vi "Format_table.vi"(2 "Table Control":refnum<vi>) -> ()   [LabVIEW 2013]
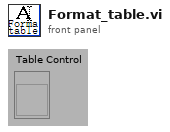
[diagram p1: front panel]
types:
  T1 = cluster{"Font Name:":string, "Size":i16, "Strikeout?":bool, "Italic?":bool, "Underline?":bool, "Outline?":bool, "Shadow?":bool, "Bold?":bool}
  T2 = enum16{"User-specified Font", "Application Font", "System Font", "Dialog Font"}
  T3 = typedef "LVFontTypeDef.ctl" = cluster{"Font Name":string, "Size":u16, "Bold":bool, "Italic":bool, "Underline":bool, "Strikeout":bool, "Color":u32}
  T4 = cluster{"left":i16, "top":i16, "right":i16, "bottom":i16}
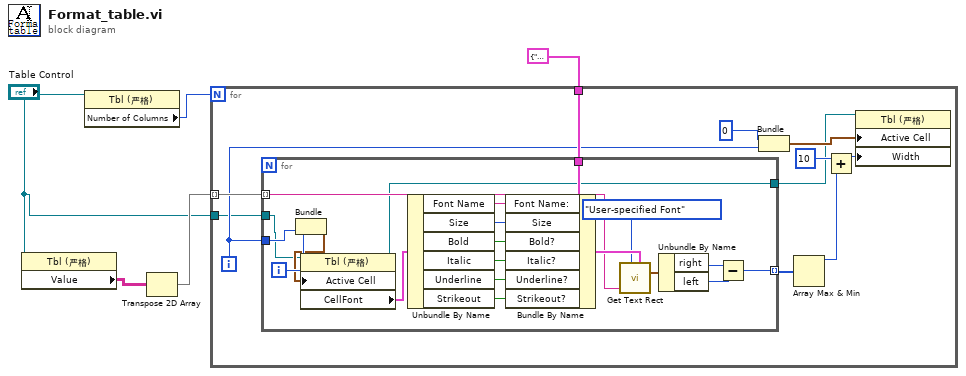
[diagram p0: block diagram]
diagram:
  n1 = property class="Tbl (严格)"(reference="Table Control") -> ("Value"=w3:string[][])  [unwired: 1 in, 2 out]
  n2 = property class="Tbl (严格)"(reference="Table Control") -> ("Number of Columns"=w2:u32)  [unwired: 1 in, 2 out]
  n3 = Transpose 2D Array(2D array=w3) -> (transposed array=w4:string[][])
  n4 = for {
    N: w2 -> [_]
    tunnel: w4 -> [w16] mode=indexing
    tunnel: T1 {"Font Name:"="", "Size"=0, "Strikeout?"=FALSE, "Italic?"=FALSE, "Underline?"=FALSE, "Outline?"=FALSE, "Shadow?"=FALSE, "Bold?"=FALSE} ("[user-specified font]") -> [w15]
    tunnel: "Table Control" -> [w7]
    i -> [w13]
    n5 = for {
      tunnel: w16 -> [w28] mode=indexing
      tunnel: w13 -> [w21]
      tunnel: w15 -> [w35]
      tunnel: [w23] -> w14 mode=indexing
      tunnel: w7 -> [w18]
      tunnel: [w17] -> w6
      i -> [w22]
      n6 = Bundle(w22, w21) -> (w20:cluster{i32, i32})  [unwired: 1 in]
      n7 = property class="Tbl (严格)"(reference=w18, "Active Cell"=w20) -> (reference out=w17:refnum<vi>, "CellFont"=w19:T3)  [unwired: 1 in, 1 out]
      n8 = Unbundle By Name(w19) -> ("Font Name"=w34:string, "Size"=w33:u16, "Bold"=w32:bool, "Italic"=w31:bool, "Underline"=w30:bool, "Strikeout"=w29:bool)
      n9 = Bundle By Name(cluster=w35, "Font Name:"=w34, "Size"=w33, "Bold?"=w32, "Italic?"=w31, "Underline?"=w30, "Strikeout?"=w29) -> (w36:T1)
      n10 = call <vilib>:"Get Text Rect.vi"("desired font(Application)"=T2."User-specified Font", "text"=w28, "[user-specified font]"=w36) -> ("rect"=w26:T4)  [unwired: 6 in]
      n11 = Unbundle By Name(w26) -> ("right"=w25:i16, "left"=w24:i16)
      n12 = Subtract(x=w25, y=w24) -> (x-y=w23:i16)
    }
    n13 = Bundle(0, w13) -> (w9:cluster{i32, i32})  [unwired: 1 in]
    n14 = Array Max & Min(array=w14) -> (max value=w10:i16)  [unwired: 3 out]
    n15 = Add(x=i16 10, y=w10) -> (x+y=w8:i16)
    n16 = property class="Tbl (严格)"(reference=w6, "Active Cell"=w9, "Width"=w8) -> ()  [unwired: 1 in, 2 out]
  }
